vi "Create Listener If Needed.vi"(5 "net address":u32, 6 "Server Alias":string, 7 "Port":u16, 8 "error in (no error)":errorcluster, 10 "Recreate?":bool, 11 "TCP Network Connection in":refnum<k5>) -> (0 "error out":errorcluster, 3 "TCP Network Connection out":refnum<k5>)   [LabVIEW 2013, in "TS.lvlib"]
doc: "This VI is the reason the LabVIEW side has to start first. The TCP Listener is on the LabVIEW side, which means we're viewing the LabVIEW side as the \"server\" in a client/server architecture. Python is the client. This VI wraps the standard Create Listener vi."
uses:
  TS.lvlib
  <vilib>/ErrorRing/Error Ring.xnode
  <vilib>/Utility/error.llb/Error Cluster From Error Code.vi
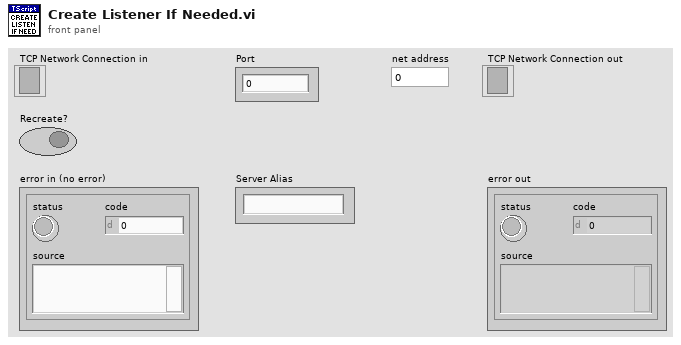
[diagram p1: front panel]
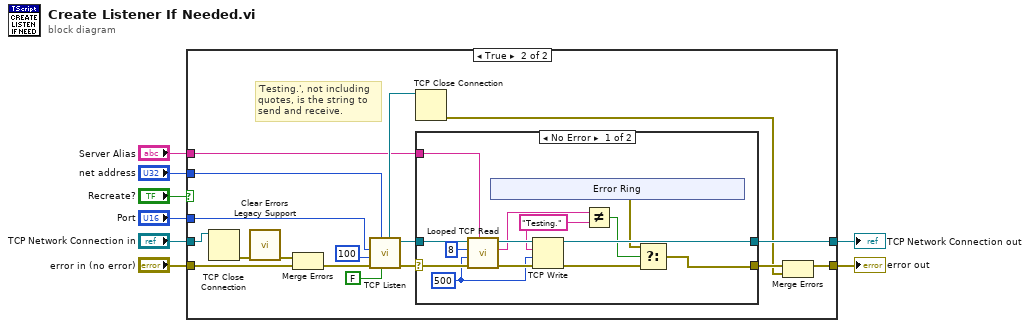
[diagram p0: block diagram]
diagram:
  n1 = case shown="True" "Recreate?" {
    tunnel: [w9 w14] -> w6
    tunnel: "error in (no error)" -> [w9 w19]
    tunnel: [w10 w24] -> w7
    tunnel: "TCP Network Connection in" -> [w10 w21]
    tunnel: "Port" -> [_ w26]
    tunnel: "net address" -> [_ w25]
    tunnel: "Server Alias" -> [_ w11]
    frame False {
    }
    frame True {
      # "'Testing.', not including\nquotes, is the string to \nsend and receive."
      n2 = TCP Close Connection(connection ID=w21) -> (error out=w20:errorcluster)  [unwired: 2 in, 1 out]
      n3 = call "Clear Errors Legacy Support.vi"("error in (no error)"=w20) -> ("error out"=w18:errorcluster)  [unwired: 5 in, 1 out]
      n4 = Merge Errors(w18, w19) -> (w17:errorcluster)
      n5 = call <vilib>:"TCP Listen.vi"("resolve remote address (T)"=FALSE, "net address"=w25, "error in (no error)"=w17, "timeout ms (wait forever: -1)"=100 ("timeout(ms)"), "port"=w26) -> ("error out"=w23:errorcluster, "connection ID"=w16:refnum<k5>, "listener ID"=w15:refnum<k5>)  [unwired: 2 in, 2 out]
      n6 = TCP Close Connection(connection ID=w15) -> (error out=w12:errorcluster)  [unwired: 2 in, 1 out]
      n7 = case shown="No Error" w23 {
        selector: w23 -> [w30 w46]
        tunnel: w16 -> [w41 w47]
        tunnel: [w37 w47] -> w24
        tunnel: [w31 w46] -> w13
        tunnel: w11 -> [w28 _]
        frame No Error {
          w35 = "Testing." ("data in")
          w29 = 500 ("timeout ms (25000)")
          n8 = call "Looped TCP Read.vi"("Server Alias"=w28, "error in (no error)"=w30, "timeout ms (25000)"=w29, "bytes to read"=8, "connection ID in"=w41) -> ("error out"=w38:errorcluster, "data out"=w36:string, "connection ID out"=w39:refnum<k5>)  [unwired: 4 in]
          n9 = xnode "Error Ring"() -> ("error out"=w32:errorcluster)
          n10 = TCP Write(connection ID=w39, data in=w35, error in (no error)=w38, 9:w29) -> (connection ID out=w37:refnum<k5>, error out=w34:errorcluster)  [unwired: 1 out]
          n11 = Not Equal?(x=w36, y=w35) -> (x != y?=w33:bool)
          n12 = Select(t=w32, s=w33, f=w34) -> (s? t:f=w31:errorcluster)
        }
        frame Error {
        }
      }
      n13 = Merge Errors(w13, w12) -> (w14:errorcluster)
    }
  }
  "TCP Network Connection out" <- w7
  "error out" <- w6
